vi "Write Outputs.vi"(8 "error in (no error)":errorcluster, 10 "Current time":timestamp, 11 "Output Sequencer in":refnum<class "Output Sequencer.lvclass">) -> (0 "error out":errorcluster, 3 "Output Sequencer out":refnum<class "Output Sequencer.lvclass">)   [LabVIEW 2020, in "Output Sequencer.lvlib" / "Output Sequencer.lvclass"]
uses:
  Output Sequencer.lvclass
  C:/Program Files/National Instruments/LabVIEW 2024/vi.lib/FlexLogger/SDK/PluginSDK.lvlibp/PEFClasses/SDK/Plugin/Plugin.lvclass
  <vilib>/FlexLogger/SDK/PluginSDK.lvlibp/PEFClasses/SDK/Plugin/DataHelpers/Write 1D DBL (NChan 1Sample).vi
  <vilib>/FlexLogger/SDK/PluginSDK.lvlibp/PEFClasses/SDK/Plugin/DataHelpers/Write 1D Bool (NChan 1 Sample).vi
  <vilib>/FlexLogger/SDK/PluginSDK.lvlibp/PEFClasses/SDK/Plugin/Plugin.lvclass
  C:/Program Files/National Instruments/LabVIEW 2024/vi.lib/FlexLogger/SDK/PluginSDK.lvlibp/PEFClasses/SDK/Processing Element/Processing Element.lvclass
  C:/Dev/GitHub/ni/niflexlogger-plugins/plugins/Output Sequencer/source/Output Sequencer/Output Sequencer/Output Sequencer.lvclass
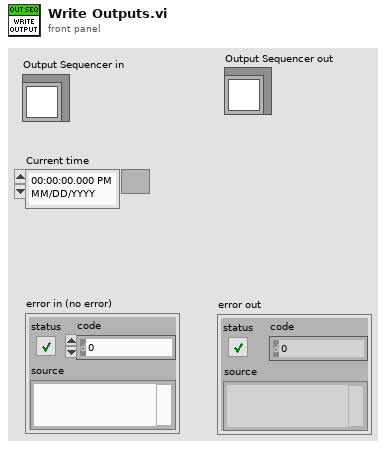
[diagram p1: front panel]
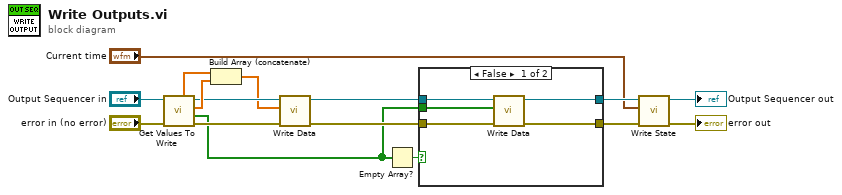
[diagram p0: block diagram]
diagram:
  n1 = call "Get Values To Write.vi"("error in (no error)"="error in (no error)", "Output Sequencer in"="Output Sequencer in") -> ("error out"=w6:errorcluster, "Digital Values to Write"=w4:bool[], "Analog Values to Write"=w14:dbl[], "Output Sequencer out"=w7:refnum<class "Output Sequencer.lvclass">, "Sequence State Channels to Write"=w15:dbl[])  [unwired: 5 in]
  n2 = Build Array (concatenate)(w15, w14) -> (w5:dbl[])
  n3 = call-poly <vilib>:"Write Data.vi"("error in (no error)"=w6, "Data"=w5, "Plugin in"=w7) -> ("error out"=w12:errorcluster, "Plugin out"=w13:refnum<class "Output Sequencer.lvclass">)  [unwired: 7 in]
  n4 = Empty Array?(array=w4) -> (empty?=w11:bool)
  n5 = case shown="False" w11 {
    tunnel: w13 -> [w21 w23]
    tunnel: w12 -> [w20 w22]
    tunnel: [w19 w23] -> w10
    tunnel: [w18 w22] -> w9
    tunnel: w4 -> [w17 _]
    frame False {
      n6 = call-poly <vilib>:"Write Data.vi"("error in (no error)"=w20, "Data"=w17, "Plugin in"=w21) -> ("error out"=w18:errorcluster, "Plugin out"=w19:refnum<class "Output Sequencer.lvclass">)  [unwired: 7 in]
    }
    frame True {
    }
  }
  n7 = call "Write State.vi"("error in (no error)"=w9, "Current time"="Current time", "Plugin in"=w10) -> ("error out"=→"error out":errorcluster, "Plugin out"=→"Output Sequencer out":refnum<class "Output Sequencer.lvclass">)  [unwired: 7 in]
